vi "Increment Pull Count.vi"(8 "error in (no error)":errorcluster, 11 "2DPanelBlank in":refnum<class "2DPanelBlank.lvclass">) -> (0 "error out":errorcluster, 3 "2DPanelBlank out":refnum<class "2DPanelBlank.lvclass">)   [LabVIEW 2020, in "OOPanel.lvlib" / "2DPanelBlank.lvclass"]
uses:
  2DPanelBlank.lvclass
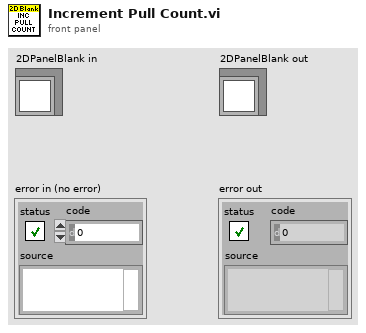
[diagram p1: front panel]
types:
  T1 = typedef "OOPanel.lvlib/2DPanelBlank.lvclass/Info.ctl" = cluster{"Index":T2, "State":T3, "Pull Count":i32}
  T2 = typedef "OOPanel.lvlib/2D Index.ctl" = cluster{"Row":i32, "Col":i32}
  T3 = typedef "OOPanel.lvlib/2DPanelBlank.lvclass/State.ctl" = enum16{"New", "Idle", "Pool", "Used", "No SP"}
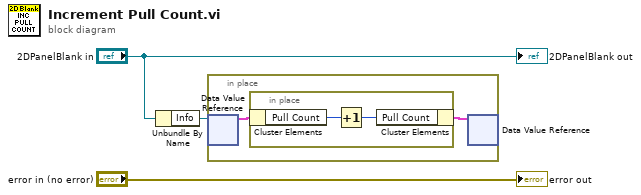
[diagram p0: block diagram]
diagram:
  n1 = Unbundle By Name("2DPanelBlank in") -> ("Info"=w2:refnum<data-value>)
  n2 = in-place {
    n3 = in-place-dvr #1(w2) -> (w5:T1)  [unwired: 1 out]
    n4 = in-place {
      n5 = in-place-cluster #2(w5) -> ("Pull Count"=w7:i32)
      n6 = Increment(x=w7) -> (x+1=w6:i32)
      n7 = in-place-cluster #2("Pull Count"=w6) -> (w4:T1)
    }
    n8 = in-place-dvr #1(w4) -> ()  [unwired: 2 out]
  }
  "error out" <- "error in (no error)"
  "2DPanelBlank out" <- "2DPanelBlank in"
